vi "To Bool Tree Data.vi"(10 "Boolean":bool) -> (3 "Bool Tree Data":refnum<class "Bool.lvclass">)   [LabVIEW 2020, in "NI_VIAnCFGDataStructure.lvlib" / "Bool.lvclass"]
doc: "Convert a Bool value to Tree Data type."
uses:
  <vilib>/addons/analyzer/VIAnCFGDataStructure/Data Types/Bool/Bool.lvclass
  <vilib>/addons/analyzer/VIAnCFGDataStructure/Data Types/Bool/Bool.lvclass/Bool.ctl
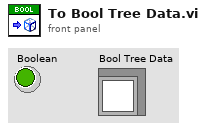
[diagram p1: front panel]
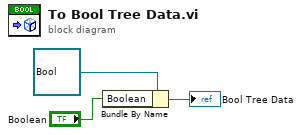
[diagram p0: block diagram]
diagram:
  n1 = Bundle By Name(cluster=refnum<class "Bool.lvclass"> refnum ("Bool in"), "Boolean"="Boolean") -> (→"Bool Tree Data":refnum<class "Bool.lvclass">)
